vi "Resolve Mapping.vi"(4 "output dictionary":refnum<class "data dictionary.lvclass">, 6 "input dictionary":refnum<class "data dictionary.lvclass">, 8 "error in":errorcluster, 10 "bitfile ref":refnum<k20>, 11 "channels in":refnum<class "TBM channel.lvclass">[](array[class])) -> (0 "error out":errorcluster, 1 "indicators":T1[](array[typedef]), 2 "controls":T1[](array[typedef]))   [LabVIEW 2017, in "FPGA Module runtime.lvclass"]
uses:
  FPGA Module runtime.lvclass
  <vilib>/NI/Tag Bus Module Framework/channel/TBM channel.lvclass
  ControlsMappings.ctl
  <vilib>/NI/Tag Bus/tag/Data Type.ctl
  fpga channel/fpga resource supported data types.ctl
  <vilib>/NI/Tag Bus/dictionary/data dictionary.lvclass
  fpga channel/FPGA Channel.lvclass
  C:/Program Files (x86)/National Instruments/LabVIEW 2017/vi.lib/NI/Tag Bus Module Framework/channel/TBM channel.lvclass
  C:/Program Files (x86)/National Instruments/LabVIEW 2017/vi.lib/NI/Tag Bus/tag/tag descriptor.lvclass
  <vilib>/NI/Tag Bus Module Framework/channel/TBM channel.lvclass/TBM channel.ctl
  <vilib>/NI/Tag Bus/tag/tag descriptor.lvclass/tag descriptor.ctl
  <vilib>/NI/Tag Bus Module Framework/channel/Read channel classification.vi
  <vilib>/NI/Tag Bus/tag/read tag name.vi
  <vilib>/NI/Tag Bus/tag/read data type.vi
  <vilib>/NI/LVFPGA Adv Session Resources/LVFPGAAdvSessionResources.lvlib
  <vilib>/NI/Tag Bus/tag/tag descriptor.lvclass
  <vilib>/NI/Configuration Framework/NISE_CEF_TreeControl.lvlib
panel:
  out "Array":string[](array[string])
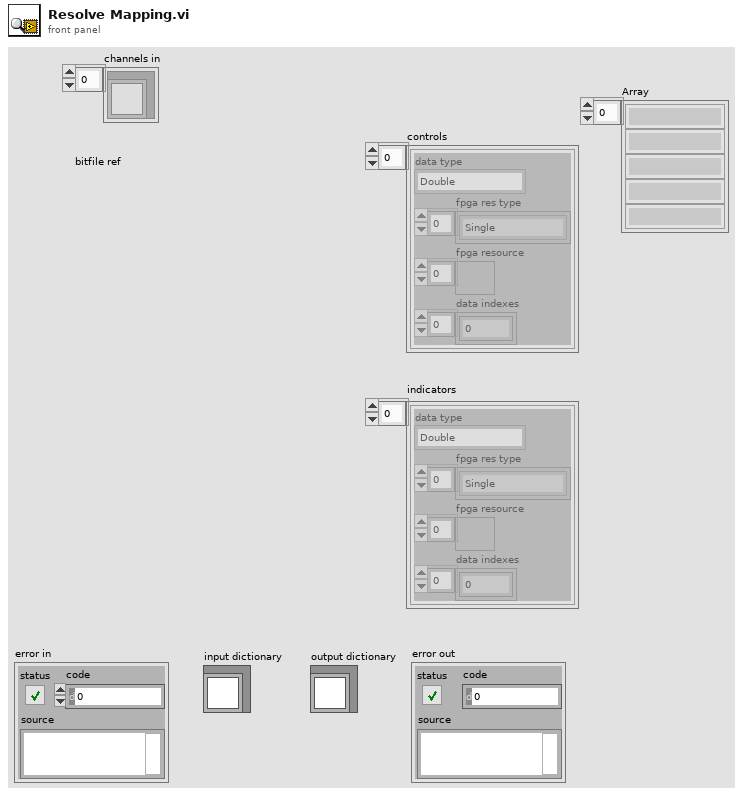
[diagram p1: front panel]
types:
  T1 = typedef "FPGA Channel.lvclass/ControlsMappings.ctl" = cluster{"data type":T2, "fpga res type":T3[], "fpga resource":refnum<k20>[], "data indexes":i32[]}
  T2 = typedef "tag bus.lvlib/tag descriptor.lvclass/Data Type.ctl" = enum16{"Double", "Single", "I64", "I32", "I16", "I8", "U64", "U32", "U16", "U8", "Boolean", "String", "Array of Double", "Array of Single", "Array of I64", "Array of I32", "Array of I16", "Array of I8", "Array of U64", "Array of U32", "Array of U16", "Array of U8", "Array of Boolean", "Array of String"}
  T3 = typedef "FPGA Channel.lvclass/fpga resource supported data types.ctl" = enum16{"Invalid Type", "Single", "I64", "I32", "I16", "I8", "U64", "U32", "U16", "U8", "Boolean", "FXP I,20,5", "FXP I,24,5", "FXP I,24,10", "Fifo 1023,I16"}
  T4 = typedef "LVFPGAAdvSessionResources.lvlib/ResourceInfo.ctl" = cluster{"Resource name":string, "Data type":variant, "Resource type":enum16{"Register", "Host To Target FIFO", "Target To Host FIFO"}}
  T5 = typedef "TBM channel.lvclass/channel classification.ctl" = enum16{"input data", "output data", "processing parameter", "processing result"}
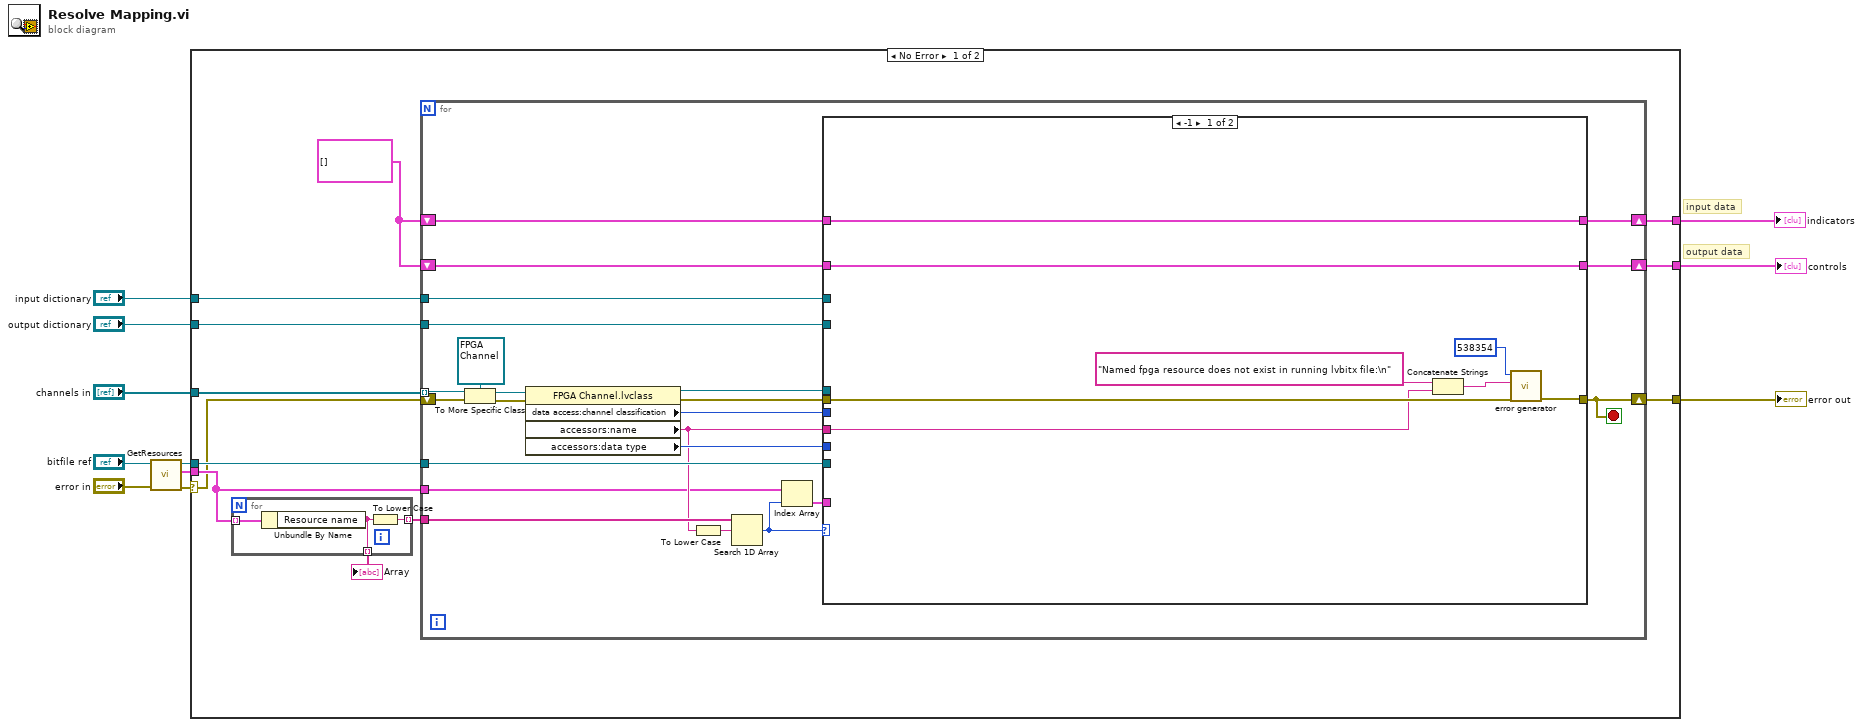
[diagram p0: block diagram]
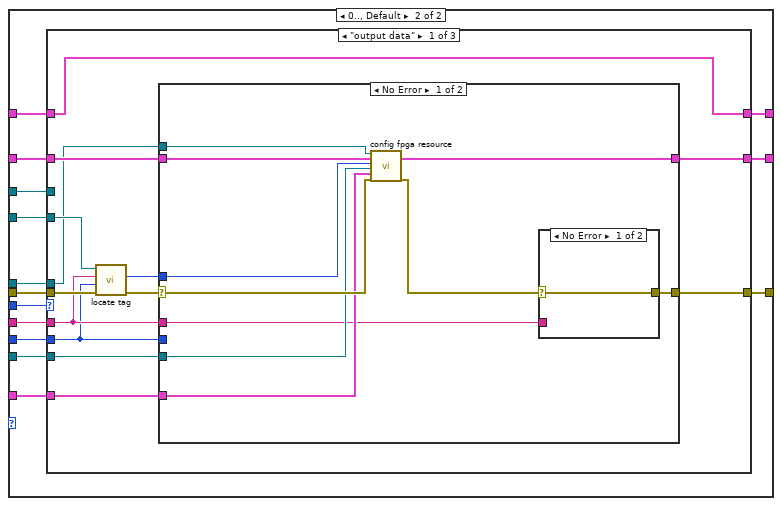
[diagram p2: hidden frame]
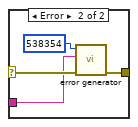
[diagram p3: hidden frame]
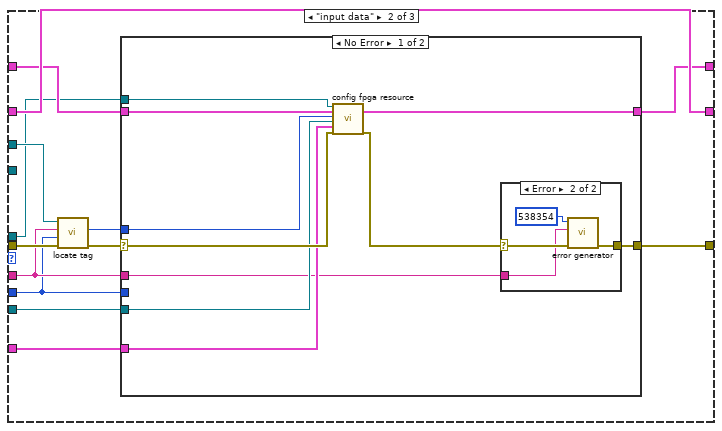
[diagram p5: hidden frame]
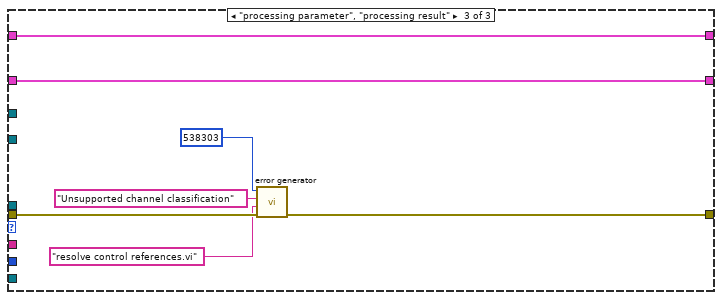
[diagram p8: hidden frame]
diagram:
  # "input data"
  # "output data"
  n1 = call <vilib>:"GetResources.vi"("error in (no error)"="error in", "FPGA VI Reference in"="bitfile ref") -> ("error out"=w1:errorcluster, "Resource info out"=w2:T4[], "FPGA VI Reference out"=w3:refnum<k20>)  [unwired: 7 in]
  n2 = case shown="No Error" w1 {
    selector: w1 -> [w14 w139]
    tunnel: "channels in" -> [w23 _]
    tunnel: [w22 _] -> w6
    tunnel: [w21 _] -> w5
    tunnel: "output dictionary" -> [w20 _]
    tunnel: "input dictionary" -> [w19 _]
    tunnel: [w18 w139] -> w7
    tunnel: w3 -> [w16 _]
    tunnel: w2 -> [w15 _]
    frame No Error {
      w13 = T1[] [] ("indicators")
      n3 = for {
        tunnel: w15 -> [w26] mode=indexing
        tunnel: [w25] -> w17 mode=indexing
        tunnel: [w24] -> w12 mode=indexing
        n4 = Unbundle By Name(w26) -> ("Resource name"=w24:string)
        n5 = To Lower Case(string=w24) -> (all lower case string=w25:string)
      }
      "Array" <- w12
      n6 = for {
        tunnel: w23 -> [w27] mode=indexing
        shift-right: [w46] -> w22
        shift-left: w13 -> [w45]
        shift-right: [w43] -> w21
        shift-left: w13 -> [w44]
        shift-right: [w47] -> w18
        shift-left: w14 -> [w34]
        tunnel: w20 -> [w41]
        tunnel: w19 -> [w42]
        tunnel: w16 -> [w40]
        tunnel: w17 -> [w37]
        tunnel: w15 -> [w30]
        stop <- w47 stop-if-true
        n7 = To More Specific Class(target class=refnum<class "FPGA Channel.lvclass"> refnum ("fpga channel.lvclass"), reference=w27, error in=w34) -> (specific class reference=w33:refnum<class "FPGA Channel.lvclass">, error out=w28:errorcluster)
        n8 = property class="FPGA Channel.lvclass"(reference=w33, error in=w28) -> (reference out=w38:refnum<class "FPGA Channel.lvclass">, error out=w48:errorcluster, "data access:channel classification"=w49:T5, "accessors:name"=w36:string, "accessors:data type"=w39:T2)
        n9 = To Lower Case(string=w36) -> (all lower case string=w35:string)
        n10 = Search 1D Array(1D array=w37, element=w35) -> (index of element=w31:i32)  [unwired: 1 in]
        n11 = Index Array(array=w30, index=w31) -> (element=w29:T4)
        n12 = case shown="-1" w31 {
          tunnel: w49 -> [_ w71]
          tunnel: w48 -> [w56 w70]
          tunnel: [w55 w69] -> w47
          tunnel: [w54 w68] -> w46
          tunnel: w45 -> [w54 w67]
          tunnel: w44 -> [w53 w66]
          tunnel: [w53 w65] -> w43
          tunnel: w42 -> [_ w64]
          tunnel: w41 -> [_ w63]
          tunnel: w40 -> [_ w62]
          tunnel: w39 -> [_ w61]
          tunnel: w38 -> [_ w60]
          tunnel: w36 -> [w50 w59]
          tunnel: w29 -> [_ w58]
          frame -1 {
            n13 = Concatenate Strings("Named fpga resource does not exist in running lvbitx file:\n" ("append error message"), w50) -> (w51:string)
            n14 = call <vilib>:"error generator.vi"("error in"=w56, "append error message"=w51, "error code (0)"=538354) -> ("error out"=w55:errorcluster)  [unwired: 6 in]
          }
          frame 0.., Default {
            n15 = case shown="\"output data\"" w71 {
              tunnel: w70 -> [w84 w113 w138]
              tunnel: [w80 w109 w136] -> w69
              tunnel: [w74 w103 w133] -> w68
              tunnel: w67 -> [w74 w104 w133]
              tunnel: w66 -> [w76 w114 w132]
              tunnel: [w75 w114 w132] -> w65
              tunnel: w64 -> [_ w105 _]
              tunnel: w59 -> [w82 w111 _]
              tunnel: w61 -> [w81 w110 _]
              tunnel: w63 -> [w77 _ _]
              tunnel: w62 -> [w78 w107 _]
              tunnel: w60 -> [w73 w102 _]
              tunnel: w58 -> [w72 w106 _]
              frame "output data" {
                n16 = call <vilib>:"locate tag.vi"("error in"=w84, "data type"=w81, "name"=w82, "data dictionary in"=w77) -> ("error out"=w83:errorcluster, "index"=w79:i32)  [unwired: 5 in, 1 out]
                n17 = case shown="No Error" w83 {
                  selector: w83 -> [w93 w101]
                  tunnel: w82 -> [w85 _]
                  tunnel: w81 -> [_ _]
                  tunnel: [w94 w101] -> w80
                  tunnel: w76 -> [w90 w100]
                  tunnel: [w89 w100] -> w75
                  tunnel: w79 -> [w88 _]
                  tunnel: w78 -> [w87 _]
                  tunnel: w73 -> [w91 _]
                  tunnel: w72 -> [w86 _]
                  frame No Error {
                    n18 = call-dynamic "config fpga resource.vi"("fpga channel in"=w91, "pairs in"=w90, "tagbus index"=w88, "bitfile ref in"=w87, "hardware resource"=w86, "error in (no error)"=w93) -> ("pairs out"=w89:T1[], "error out"=w92:errorcluster)  [unwired: 11 in, 1 out]
                    n19 = case shown="No Error" w92 {
                      selector: w92 -> [w95 w97]
                      tunnel: [w95 w98] -> w94
                      tunnel: w85 -> [_ w96]
                      frame No Error {
                      }
                      frame Error {
                        n20 = call <vilib>:"error generator.vi"("error in"=w97, "append error message"=w96, "error code (0)"=538354) -> ("error out"=w98:errorcluster)  [unwired: 6 in]
                      }
                    }
                  }
                  frame Error {
                  }
                }
              }
              frame "input data" {
                n21 = call <vilib>:"locate tag.vi"("error in"=w113, "data type"=w110, "name"=w111, "data dictionary in"=w105) -> ("error out"=w112:errorcluster, "index"=w108:i32)  [unwired: 5 in, 1 out]
                n22 = case shown="No Error" w112 {
                  selector: w112 -> [w123 w131]
                  tunnel: w111 -> [w115 _]
                  tunnel: w110 -> [_ _]
                  tunnel: [w124 w131] -> w109
                  tunnel: w104 -> [w120 w130]
                  tunnel: [w119 w130] -> w103
                  tunnel: w108 -> [w118 _]
                  tunnel: w107 -> [w117 _]
                  tunnel: w102 -> [w121 _]
                  tunnel: w106 -> [w116 _]
                  frame No Error {
                    n23 = call-dynamic "config fpga resource.vi"("fpga channel in"=w121, "pairs in"=w120, "tagbus index"=w118, "bitfile ref in"=w117, "hardware resource"=w116, "error in (no error)"=w123) -> ("pairs out"=w119:T1[], "error out"=w122:errorcluster)  [unwired: 11 in, 1 out]
                    n24 = case shown="Error" w122 {
                      selector: w122 -> [w125 w127]
                      tunnel: [w125 w128] -> w124
                      tunnel: w115 -> [_ w126]
                      frame No Error {
                      }
                      frame Error {
                        n25 = call <vilib>:"error generator.vi"("error in"=w127, "append error message"=w126, "error code (0)"=538354) -> ("error out"=w128:errorcluster)  [unwired: 6 in]
                      }
                    }
                  }
                  frame Error {
                  }
                }
              }
              frame "processing parameter", "processing result" {
                n26 = call <vilib>:"error generator.vi"("error in"=w138, "source"="resolve control references.vi", "append error message"="Unsupported channel classification", "error code (0)"=538303) -> ("error out"=w136:errorcluster)  [unwired: 5 in]
              }
            }
          }
        }
      }
    }
    frame Error {
    }
  }
  "controls" <- w5
  "indicators" <- w6
  "error out" <- w7
